vi "CreatRegedit.vi"(8 "error in":errorcluster caption="错误输入（无错误）", 9 "值":string[](array[string]), 10 "名称":string[](array[string]), 11 "subkey":string="SuperJoint\\MyKey") -> (0 "error out":errorcluster caption="错误输出")   [LabVIEW 2018]
uses:
  <vilib>/registry/registry.llb/Registry RtKey.ctl
  <vilib>/registry/registry.llb/Write Registry Value Simple STR.vi
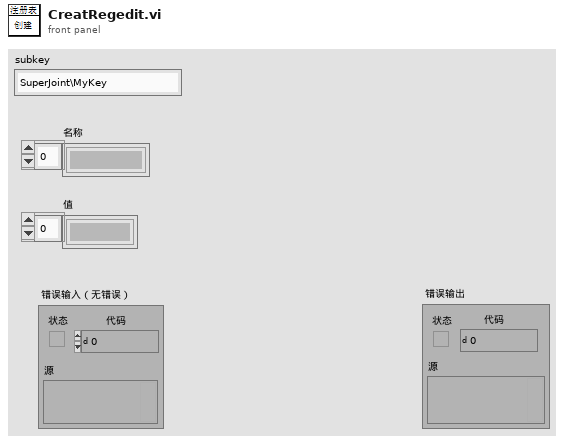
[diagram p1: front panel]
types:
  T1 = typedef "Registry RtKey.ctl" = enum32{"HKEY_CLASSES_ROOT", "HKEY_CURRENT_USER", "HKEY_LOCAL_MACHINE", "HKEY_USERS", "HKEY_PERFORMANCE_DATA", "HKEY_CURRENT_CONFIG", "HKEY_DYN_DATA"}
  T2 = typedef "Registry refnum.ctl" = refnum<k1>
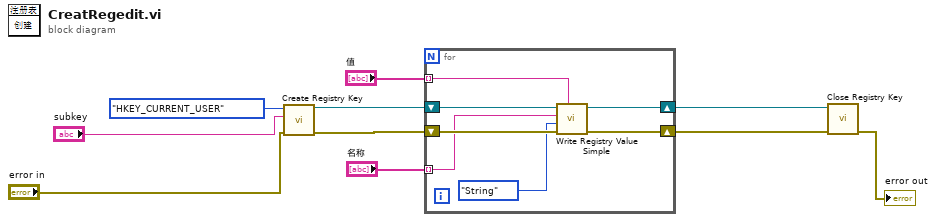
[diagram p0: block diagram]
diagram:
  n1 = call <vilib>:"Create Registry Key.vi"("error in (no error)"="error in", "subkey"="subkey", "root key (HKEY_LOCAL_MACHINE)"=Registry_RtKey."HKEY_CURRENT_USER") -> ("error out"=w7:errorcluster, "refnum out"=w8:T2)  [unwired: 6 in, 1 out]
  n2 = for {
    shift-right: [w14] -> w5
    shift-left: w8 -> [w17]
    shift-right: [w15] -> w6
    shift-left: w7 -> [w16]
    tunnel: "值" -> [w12] mode=indexing
    tunnel: "名称" -> [w11] mode=indexing
    n3 = call-poly <vilib>:"Write Registry Value Simple.vi"("String/Binary data"=w12, "error in (no error)"=w16, "simple data type"=enum16{"String", "Binary", "DWORD"}."String", "value"=w11, "refnum"=w17) -> ("error out"=w15:errorcluster, "refnum out"=w14:T2)  [unwired: 3 in]
  }
  n4 = call <vilib>:"Close Registry Key.vi"("error in (no error)"=w6, "refnum"=w5) -> ("error out"=→"error out":errorcluster)  [unwired: 5 in]
